vi "Write Allow Undefinded Values.vi"(5 "Allow Undefinded Values":bool, 9 "Ring in":refnum<class "Ring.lvclass">) -> (3 "Ring out":refnum<class "Ring.lvclass">)   [LabVIEW 2014, in "Raspberry Pi Compatible Compiler for LabVIEW.lvlib" / "Ring.lvclass"]
uses:
  Ring.lvclass
  Ring.lvclass/Ring.ctl
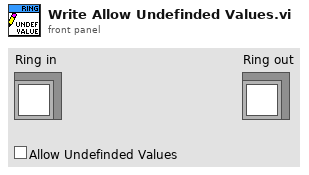
[diagram p1: front panel]
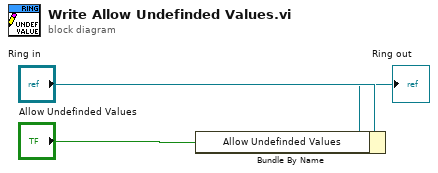
[diagram p0: block diagram]
diagram:
  n1 = Bundle By Name(cluster="Ring in", "Allow Undefinded Values"="Allow Undefinded Values") -> (→"Ring out":refnum<class "Ring.lvclass">)
